vi "runTestScenario.vi"(0 "ITestScenario in":refnum<class "NotImplementedTest.lvclass">, 5 "ILC":refnum<class "ILC.lvclass">, 11 "error in (no error)":errorcluster) -> (4 "ITestScenario out":refnum<class "NotImplementedTest.lvclass">, 6 "ILC 2":refnum<class "ILC.lvclass">, 8 "TestExecution":T2, 10 "Result":T1, 15 "error out":errorcluster)   [LabVIEW 2015, in "NotImplementedTest.lvclass"]
uses:
  NotImplementedTest.lvclass
  Typedefs/TestExecution.ctl
  Typedefs/PassFailTest.ctl
  <userlib>/Common/ILC/ILC/ILC.lvclass
  Typedefs/ILCBTTypedefs.lvlib
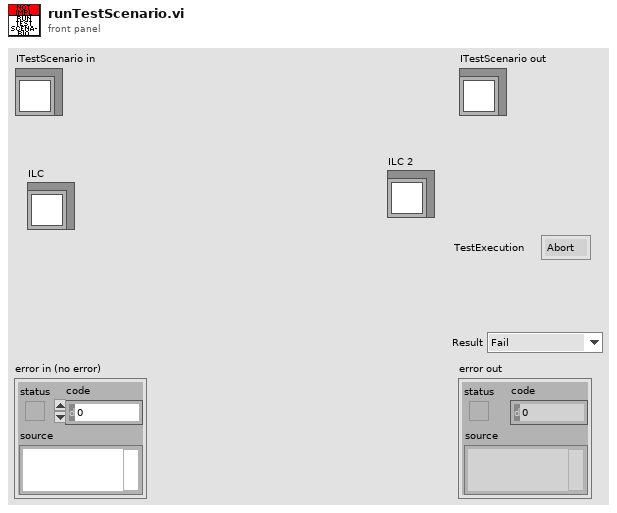
[diagram p1: front panel]
types:
  T1 = typedef "ILCBTTypedefs.lvlib/PassFailTest.ctl" = enum16{"Fail", "Pass", "NA"}
  T2 = typedef "ILCBTTypedefs.lvlib/TestExecution.ctl" = enum16{"Abort", "Continue"}
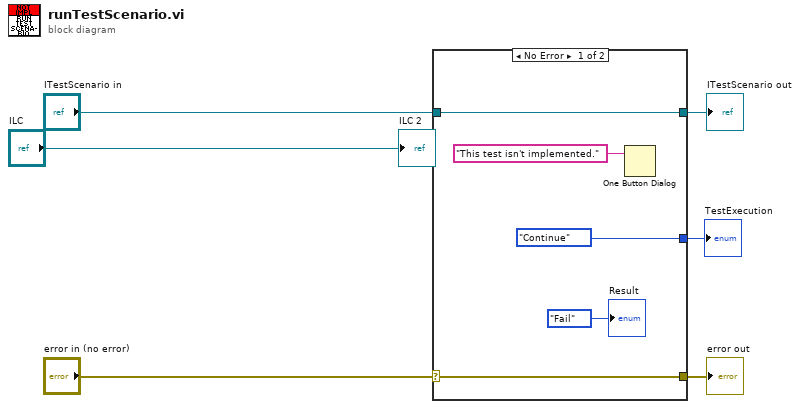
[diagram p0: block diagram]
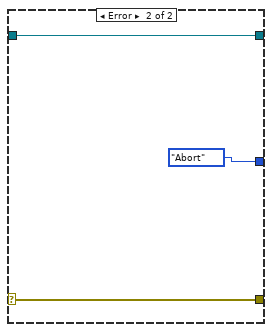
[diagram p2: hidden frame]
diagram:
  n1 = case shown="No Error" "error in (no error)" {
    selector: "error in (no error)" -> [w10 w14]
    tunnel: [w10 w14] -> w5
    tunnel: [w11 w13] -> w3
    tunnel: "ITestScenario in" -> [w11 w13]
    tunnel: [TestExecution."Continue" ("TestExecution") TestExecution."Abort" ("TestExecution")] -> w2
    frame No Error {
      n2 = One Button Dialog(message="This test isn't implemented.") -> ()  [unwired: 1 in, 1 out]
      "Result" <- PassFailTest."Fail" ("Result")
    }
    frame Error {
    }
  }
  "error out" <- w5
  "ITestScenario out" <- w3
  "TestExecution" <- w2
  "ILC 2" <- "ILC"
